vi "GetCartesianPosition.vi"(0 "error in (no error)":errorcluster, 7 "HighSpeedEServer":refnum<k24>) -> (4 "error out":errorcluster, 6 "Pose":T1, 8 "RCONF":i32, 10 "ToolNumber":i32, 15 "UserCoordinateNumber":i32)   [LabVIEW 2012, in "UnderAutomation.Yaskawa.lvlib"]
uses:
  UnderAutomation.Yaskawa.lvlib
  C:/Users/fg/Documents/Yaskawa.vi/LabVIEW_2024/UnderAutomation.Yaskawa/lib/UnderAutomation.Yaskawa.dll
  LabVIEW_2024/UnderAutomation.Yaskawa/lib/UnderAutomation.Yaskawa.dll
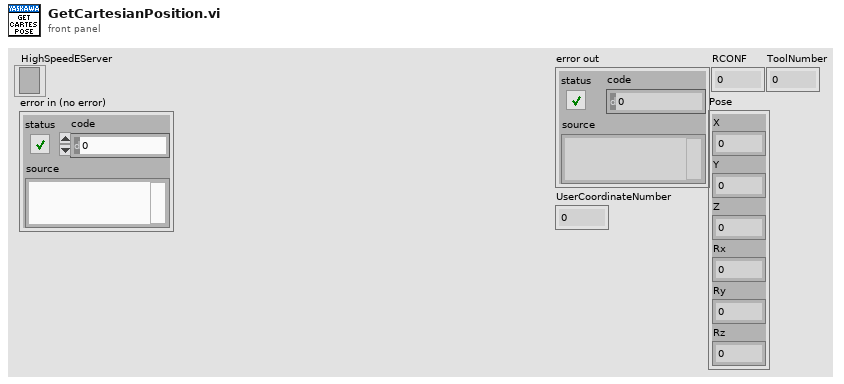
[diagram p1: front panel]
types:
  T1 = cluster{"X":dbl, "Y":dbl, "Z":dbl, "Rx":dbl, "Ry":dbl, "Rz":dbl}
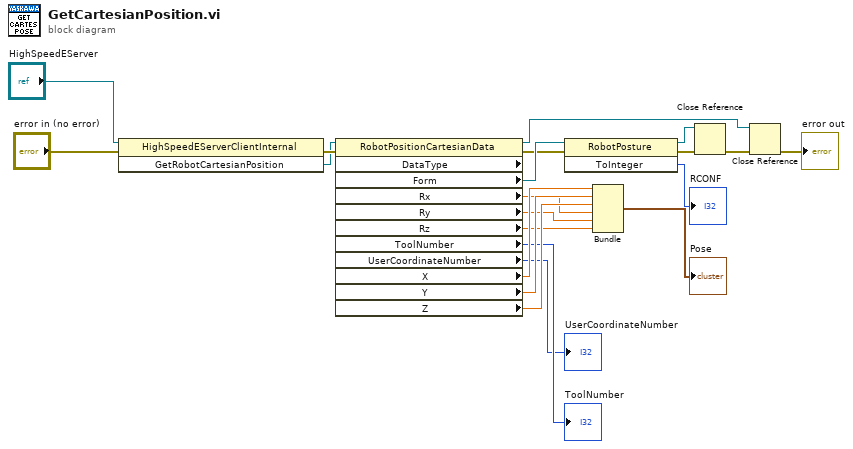
[diagram p0: block diagram]
diagram:
  n1 = invoke class="HighSpeedEServerClientInternal" method="GetRobotCartesianPosition"(reference="HighSpeedEServer", error in="error in (no error)") -> (error out=w19:errorcluster, "GetRobotCartesianPosition"=w18:refnum<k24>)  [unwired: 1 in, 1 out]
  n2 = property class="RobotPositionCartesianData" props=["DataType", "Form", "Rx", "Ry", "Rz", "ToolNumber", "UserCoordinateNumber", "X", "Y", "Z"](reference=w18, error in=w19) -> (reference out=w1:refnum<k24>, error out=w16:errorcluster, "Form"=w17:refnum<k24>, "Rx"=w12:dbl, "Ry"=w11:dbl, "Rz"=w10:dbl, "ToolNumber"=→"ToolNumber":i32, "UserCoordinateNumber"=→"UserCoordinateNumber":i32, "X"=w15:dbl, "Y"=w14:dbl, "Z"=w13:dbl)  [unwired: 1 out]
  n3 = invoke class="RobotPosture" method="ToInteger"(reference=w17, error in=w16) -> (reference out=w2:refnum<k24>, error out=w3:errorcluster, "ToInteger"=→"RCONF":i32)  [unwired: 1 in]
  n4 = Bundle("X"=w15, "Y"=w14, "Z"=w13, "Rx"=w12, "Ry"=w11, "Rz"=w10) -> (→"Pose":T1)  [unwired: 1 in]
  n5 = Close Reference(reference=w2, error in (no error)=w3) -> (error out=w4:errorcluster)
  n6 = Close Reference(reference=w1, error in (no error)=w4) -> (error out=→"error out":errorcluster)
